vi "check focus or flystart.vi"(11 "x":string) -> (3 "x .or. y?":bool)   [LabVIEW 2012]
uses:
  GFG/GFGbooleanGet.vi
  GFG/GFG library.lvlib
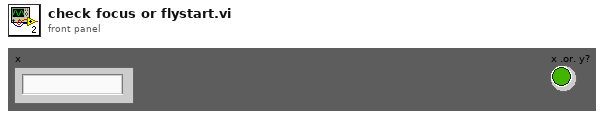
[diagram p1: front panel]
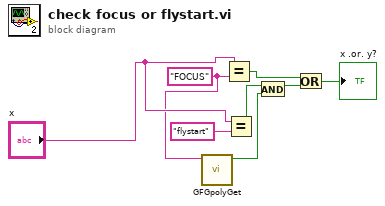
[diagram p0: block diagram]
diagram:
  w1 = "FOCUS" ("y")
  n1 = call-poly "GFGpolyGet.vi"("Variable Name in"=w1) -> ("Boolean"=w4:bool)  [unwired: 10 in]
  n2 = Equal?(x="x", y=w1) -> (x = y?=w8:bool)
  n3 = Equal?(x="x", y="flystart") -> (x = y?=w6:bool)
  n4 = And(x=w6, y=w4) -> (x .and. y?=w5:bool)
  n5 = Or(x=w8, y=w5) -> (x .or. y?=→"x .or. y?":bool)
